vi "Launch from TCP.vi"(8 "URI":refnum<class "URI.lvclass">, 9 "TCP Connection":refnum<k5>, 10 "Server Endpoint":refnum<class "Endpoint.lvclass">, 11 "Listener Notifier":refnum<notifier>) -> (0 "error out":errorcluster)   [LabVIEW 2020, in "Stream-Websocket.lvlib" / "Websocket Client.lvclass"]
uses:
  Websocket Client.lvclass
  lv-stream/stream/URI/URI.lvclass
  Listener Result.ctl
  Listener Status.ctl
  lv-stream/stream/Endpoint/Endpoint.lvclass
  From TCP Async.vi
  Stream-Websocket.lvlib
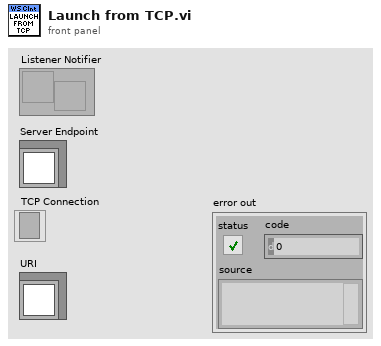
[diagram p1: front panel]
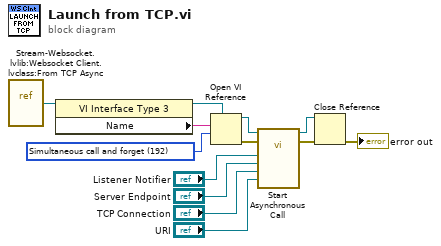
[diagram p0: block diagram]
diagram:
  w8 = 192 items=["Record modifications"=1, "Open templates for editing"=2, "Prompt user to save"=4, "Prepare for reentrant run"=8, "Prompt to find missing subVIs"=16, "Hide loading dialog box"=32, "Enable simultaneous calls"=64, "Prepare to call and forget"=128, "Simultaneous call and forget"=192, "Prepare to call and collect"=256, "Simultaneous call and collect"=320]
  n1 = vi-ref "Stream-Websocket.lvlib:Websocket Client.lvclass:From TCP Async.vi"() -> (w6:refnum<vi>)
  n2 = property class="VI Interface Type 3"(reference=w6) -> (reference out=w9:refnum<vi>, "Name"=w7:string)  [unwired: 1 in, 1 out]
  n3 = Open VI Reference(type specifier VI Refnum (for type only)=w9, vi path=w7, options=w8) -> (vi reference=w11:refnum<vi>, error out=w10:errorcluster)  [unwired: 3 in]
  n4 = call-by-ref "Start Asynchronous Call"(reference=w11, error in=w10, "URI"="URI", "TCP"="TCP Connection", "Server Endpoint"="Server Endpoint", "Listener Notifier"="Listener Notifier") -> (reference out=w13:refnum<vi>, error out=w12:errorcluster)  [unwired: 8 in]
  n5 = Close Reference(reference=w13, error in (no error)=w12) -> (error out=→"error out":errorcluster)
